vi "Calibrate Sensor Angle.vi"() -> ()   [LabVIEW 2011]
uses:
  <vilib>/robotics/Starter Kit/1.0/9631 Host Interface/NI_Robotics_Starter Kit Host_9631_1.0.lvclass
  <vilib>/Utility/AngleManip/Degrees to Radians (Scalar DBL).vi
  <vilib>/Utility/AngleManip/NI_AngleManipulation.lvlib
  <vilib>/robotics/Starter Kit/Host Interface/NI_Robotics_Starter Kit Host.lvclass
panel:
  in  "sensor motor angle":dbl(slide) caption="Sensor Motor Angle (degrees)" scale=90.0..-90.0
  in  "zero":bool
  in  "stop":bool
  # "Adjust the slider until the sensor is facing directly forward on the robot, then press Zero Angle to calibrate the sensor orientation."
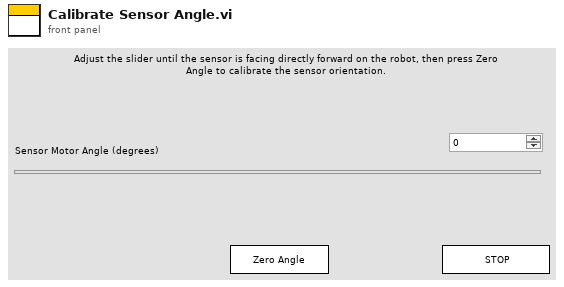
[diagram p1: front panel]
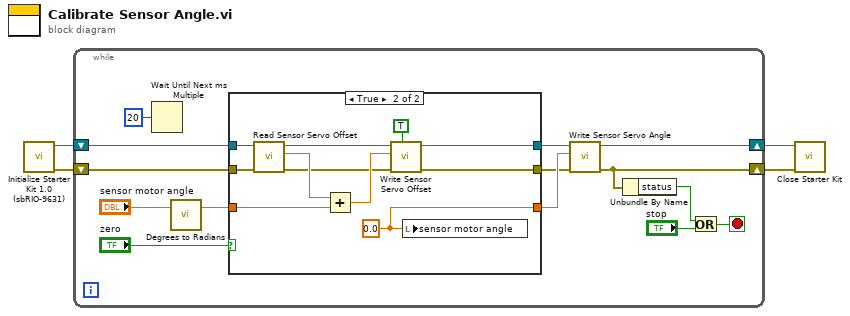
[diagram p0: block diagram]
diagram:
  n1 = call <vilib>:"Initialize Starter Kit 1.0 (sbRIO-9631).vi"() -> ("error out"=w3:errorcluster, "FPGA starter kit host 1.0 out"=w4:refnum<class "NI_Robotics_Starter Kit Host_9631_1.0.lvclass">)  [unwired: 10 in]
  n2 = while {
    shift-right: [w5] -> w2
    shift-left: w4 -> [w13]
    shift-right: [w8] -> w1
    shift-left: w3 -> [w14]
    stop <- w17 stop-if-true
    n3 = Wait Until Next ms Multiple(millisecond multiple=u32 20) -> ()  [unwired: 1 out]
    n4 = call-poly <vilib>:"Degrees to Radians.vi"("angle (deg)"="sensor motor angle") -> ("angle (rad)"=w10:dbl)  [unwired: 2 in]
    n5 = case shown="True" "zero" {
      tunnel: w14 -> [w20 w23]
      tunnel: w13 -> [w21 w24]
      tunnel: [w21 w27] -> w7
      tunnel: [w20 w25] -> w6
      tunnel: w10 -> [w19 w31]
      tunnel: [w19 w32] -> w9
      frame False {
      }
      frame True {
        w32 = 0.0 ("sensor motor angle")
        n6 = call <vilib>:"Read Sensor Servo Offset.vi"("error in (no error)"=w23, "starter kit host in"=w24) -> ("error out"=w22:errorcluster, "ccw offset angle (rad)"=w30:dbl, "starter kit host out"=w28:refnum<class "NI_Robotics_Starter Kit Host_9631_1.0.lvclass">)  [unwired: 7 in]
        n7 = Add(x=w30, y=w31) -> (x+y=w29:dbl)
        n8 = call <vilib>:"Write Sensor Servo Offset.vi"("save to file (F)"=TRUE, "error in (no error)"=w22, "ccw offset angle (rad)"=w29, "starter kit host in"=w28) -> ("error out"=w25:errorcluster, "starter kit host out"=w27:refnum<class "NI_Robotics_Starter Kit Host_9631_1.0.lvclass">)  [unwired: 6 in]
        n9 = local write "sensor motor angle"(w32) -> ()
      }
    }
    n10 = call <vilib>:"Write Sensor Servo Angle.vi"("error in (no error)"=w6, "ccw servo angle (rad)"=w9, "starter kit host in"=w7) -> ("error out"=w8:errorcluster, "starter kit host out"=w5:refnum<class "NI_Robotics_Starter Kit Host_9631_1.0.lvclass">)  [unwired: 7 in]
    n11 = Unbundle By Name(w8) -> ("status"=w16:bool)
    n12 = Or(x=w16, y="stop") -> (x .or. y?=w17:bool)
  }
  n13 = call-dynamic "Close Starter Kit.vi"("error in (no error)"=w1, "starter kit host in"=w2) -> ()  [unwired: 9 in, 1 out]
